vi "Manual open close init image.vi"(8 "error in (no error)":errorcluster, 11 "Function\ncommand":string) -> (0 "error out":errorcluster)   [LabVIEW 2019, in "ZenGage v3.0 UI.lvclass"]
uses:
  ZenGage v3.0 UI.lvclass
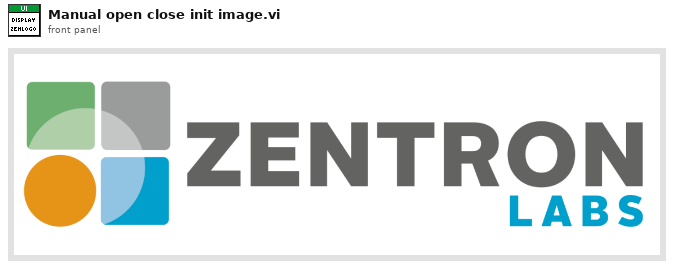
[diagram p1: front panel]
types:
  T1 = enum32{"Invalid", "Standard", "Closed", "Hidden", "Minimized", "Maximized"}
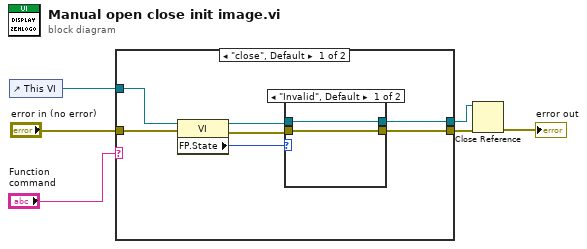
[diagram p0: block diagram]
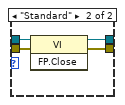
[diagram p2: hidden frame]
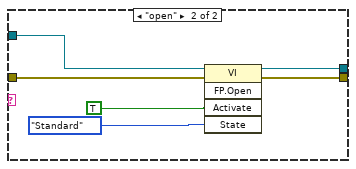
[diagram p3: hidden frame]
diagram:
  n1 = control-ref of="This VI"() -> (w5:refnum<vi>)
  n2 = case shown="\"close\", Default" "Function\ncommand" {
    tunnel: w5 -> [w9 w25]
    tunnel: "error in (no error)" -> [w11 w24]
    tunnel: [w13 w23] -> w3
    tunnel: [w12 w20] -> w1
    frame "close", Default {
      n3 = property class="VI"(reference=w9, error in=w11) -> (reference out=w8:refnum<vi>, error out=w10:errorcluster, "FP.State"=w7:T1)
      n4 = case shown="\"Invalid\", Default" w7 {
        tunnel: w10 -> [w14 w19]
        tunnel: [w14 w18] -> w13
        tunnel: w8 -> [w15 w17]
        tunnel: [w15 w16] -> w12
        frame "Invalid", Default {
        }
        frame "Standard" {
          n5 = invoke class="VI" method="FP.Close"(reference=w17, error in=w19) -> (reference out=w16:refnum<vi>, error out=w18:errorcluster)  [unwired: 1 in, 1 out]
        }
      }
    }
    frame "open" {
      n6 = invoke class="VI" method="FP.Open"(reference=w25, error in=w24, "Activate"=TRUE ("Activate?"), "State"=T1."Standard") -> (reference out=w20:refnum<vi>, error out=w23:errorcluster)  [unwired: 1 in, 3 out]
    }
  }
  n7 = Close Reference(reference=w1, error in (no error)=w3) -> (error out=→"error out":errorcluster)
